vi "Rio_Main.vi"() -> ()   [LabVIEW 2017]
doc: "The myRIO Project template acquires acceleration data from the onboard accelerometer and displays the changes of acceleration values in a waveform chart."
uses:
  rio_states.ctl
  <vilib>/myRIO/Common/Instrument Driver Framework/myRIO v1.0/Encoder/typedefs/Encoder Signal Mode.ctl
  <vilib>/myRIO/Instrument Drivers/Onboard IO/Encoder/typedefs/Encoder Reference.ctl
  <vilib>/myRIO/Common/Instrument Driver Framework/Utilities/typedefs/myRIO Generic Hardware Reference.ctl
  <vilib>/myRIO/Common/Instrument Driver Framework/Utilities/typedefs/Hardware Version Enum.ctl
  <vilib>/myRIO/Common/Instrument Driver Framework/Utilities/typedefs/myRIO v1.0 Reference.ctl
  <vilib>/myRIO/Common/Instrument Driver Framework/Utilities/typedefs/Generic FPGA Reference.ctl
  <vilib>/myRIO/Common/Instrument Driver Framework/myRIO v1.0/Encoder/typedefs/Encoder Channels Enum.ctl
  <vilib>/myRIO/Common/Instrument Driver Framework/myRIO v1.0/Encoder/typedefs/Encoder Configuration v1.0.ctl
  <vilib>/userdefined/High Color/nirio_resource_hc.ctl
  <vilib>/myRIO/Common/Instrument Driver Framework/Utilities/vis/Is FPGA Ref Available.vi
  <vilib>/myRIO/Common/Instrument Driver Framework/myRIO v1.0/Encoder/vis/myRIO v1.1 Open Encoder.vi
  <vilib>/myRIO/Instrument Drivers/Onboard IO/Encoder/vis/Read.vi
  <vilib>/myRIO/Common/Instrument Driver Framework/Utilities/vis/Validate Channels.vi
  <vilib>/myRIO/Common/Instrument Driver Framework/myRIO v1.0/Encoder/vis/myRIO v1.0 Reserve Encoder.vi
  <vilib>/myRIO/Common/Instrument Driver Framework/myRIO v1.0/Encoder/vis/myRIO v1.0 Build MUX Configuration Encoder.vi
  <vilib>/myRIO/Common/Instrument Driver Framework/myRIO v1.0/Resource Manager/vis/myRIO v1.0 Reserve Channel List.vi
  <vilib>/myRIO/Common/Instrument Driver Framework/myRIO v1.0/Resource Manager/vis/myRIO v1.0 Create Configuration List.vi
  <vilib>/myRIO/Common/Instrument Driver Framework/myRIO v1.0/Resource Manager/vis/myRIO v1.0 Reserve Channel.vi
  <vilib>/myRIO/Common/Instrument Driver Framework/myRIO v1.0/Resource Manager/vis/myRIO v1.0 Unreserve Channel.vi
  <vilib>/myRIO/Common/Instrument Driver Framework/myRIO v1.0/Resource Manager/vis/myRIO v1.0 Build Mutex Name.vi
  <vilib>/Utility/VariantDataType/GetNumericInfo.vi
  <vilib>/Utility/error.llb/Error Cluster From Error Code.vi
  <vilib>/myRIO/Common/Instrument Driver Framework/myRIO v1.0/myRIO v1.1 Open.vi
  <vilib>/myRIO/Common/Instrument Driver Framework/Utilities/vis/IO Manager.vi
  <vilib>/myRIO/Common/Instrument Driver Framework/Utilities/vis/Configuration Manager.vi
  <vilib>/myRIO/Common/Instrument Driver Framework/myRIO v1.0/Resource Manager/vis/myRIO v1.0 Configure IO.vi
  <vilib>/myRIO/Common/Instrument Driver Framework/myRIO v1.0/myRIO v1.0 Close.vi
  <vilib>/myRIO/Common/Instrument Driver Framework/myRIO v1.0/Encoder/vis/myRIO v1.0 Configure Encoder.vi
  <vilib>/myRIO/Common/Instrument Driver Framework/myRIO v1.0/Encoder/vis/myRIO v1.0 Read Encoder.vi
  <vilib>/myRIO/Express VI/Onboard IO/Encoder/Encoder Express VI.xnode
  <vilib>/myRIO/Instrument Drivers/Onboard IO/Encoder/vis/myRIO Encoder Open.xnode
  <vilib>/myRIO/Common/Instrument Driver Framework/myRIO v1.0/Encoder/typedefs/Encoder Count Direction Enum.ctl
  <vilib>/myRIO/Instrument Drivers/Onboard IO/Encoder/Encoder.lvlib
panel:
  in  "Array":dbl[][](array[numeric]) format="%#_13g"
  in  "stop":bool
  out "Y Encoder":i32
  out "Y Encoder":i32
  in  "rio_states":T1
  out "String":string
  in  "Calibrate XY":bool
  out "Error Out":errorcluster
  in  "Error In":errorcluster
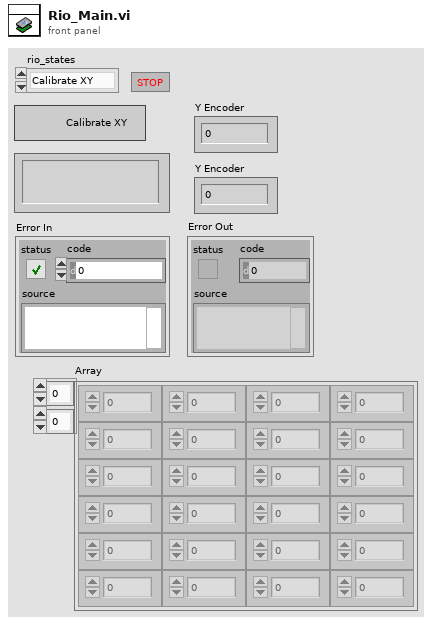
[diagram p1: front panel]
types:
  T1 = typedef "rio_states.ctl" = enum16{"Calibrate XY", "Move Theta", "Move XY", "Collect Kicker", "Pickup Kicker", "Retract Kicker", "Hold Kicker", "Kick", "Return Home", "Next Shot", "Stop"}
  T2 = typedef "rio_states.ctl" = cluster{enum16{"Calibrate XY", "Calibrate Theta", "Pickup Kicker", "Raise Kicker", "Move XY", "Move Theta", "Set Kicker Power", "Kick", "Stop"}, "Message Data":variant}
  T3 = enum16{"Calibrate XY", "Calibrate Theta", "Pickup Kicker", "Raise Kicker", "Move XY", "Move Theta", "Set Kicker Power", "Kick", "Stop"}
  T4 = typedef "Encoder.lvlib/Encoder Reference.ctl" = cluster{"myRIO Reference":T5, "Encoder Channels Enum":T9}
  T5 = typedef "myRIO Generic Hardware Reference.ctl" = cluster{"myRIO Model":T6, "myRIO Hardware Reference":T7}
  T6 = typedef "Hardware Version Enum.ctl" = enum16{"Unknown", "myRIO-1900", "myRIO-1950", "roboRIO", "NI ELVIS RIO CM"}
  T7 = typedef "myRIO v1.0 Reference.ctl" = cluster{"Generic FPGA Reference":T8, "Allow multiple opens":bool}
  T8 = typedef "Generic FPGA Reference.ctl" = refnum<k20>
  T9 = typedef "Encoder Channels Enum.ctl" = enum16{"Not Connected", "C/ENC0", "C/ENC1", "A/ENC", "B/ENC", "DIO/ENC0", "DIO/ENC1", "DIO/ENC2", "DIO/ENC3", "DIO/ENC4"}
  T10 = typedef "Encoder Signal Mode.ctl" = enum16{"Quadrature phase signal", "Step and direction signal"}
  T11 = typedef "nirio_resource_hc.ctl" = tag
  T12 = cluster{"Counter Value":i32, "Counter Value":i32}
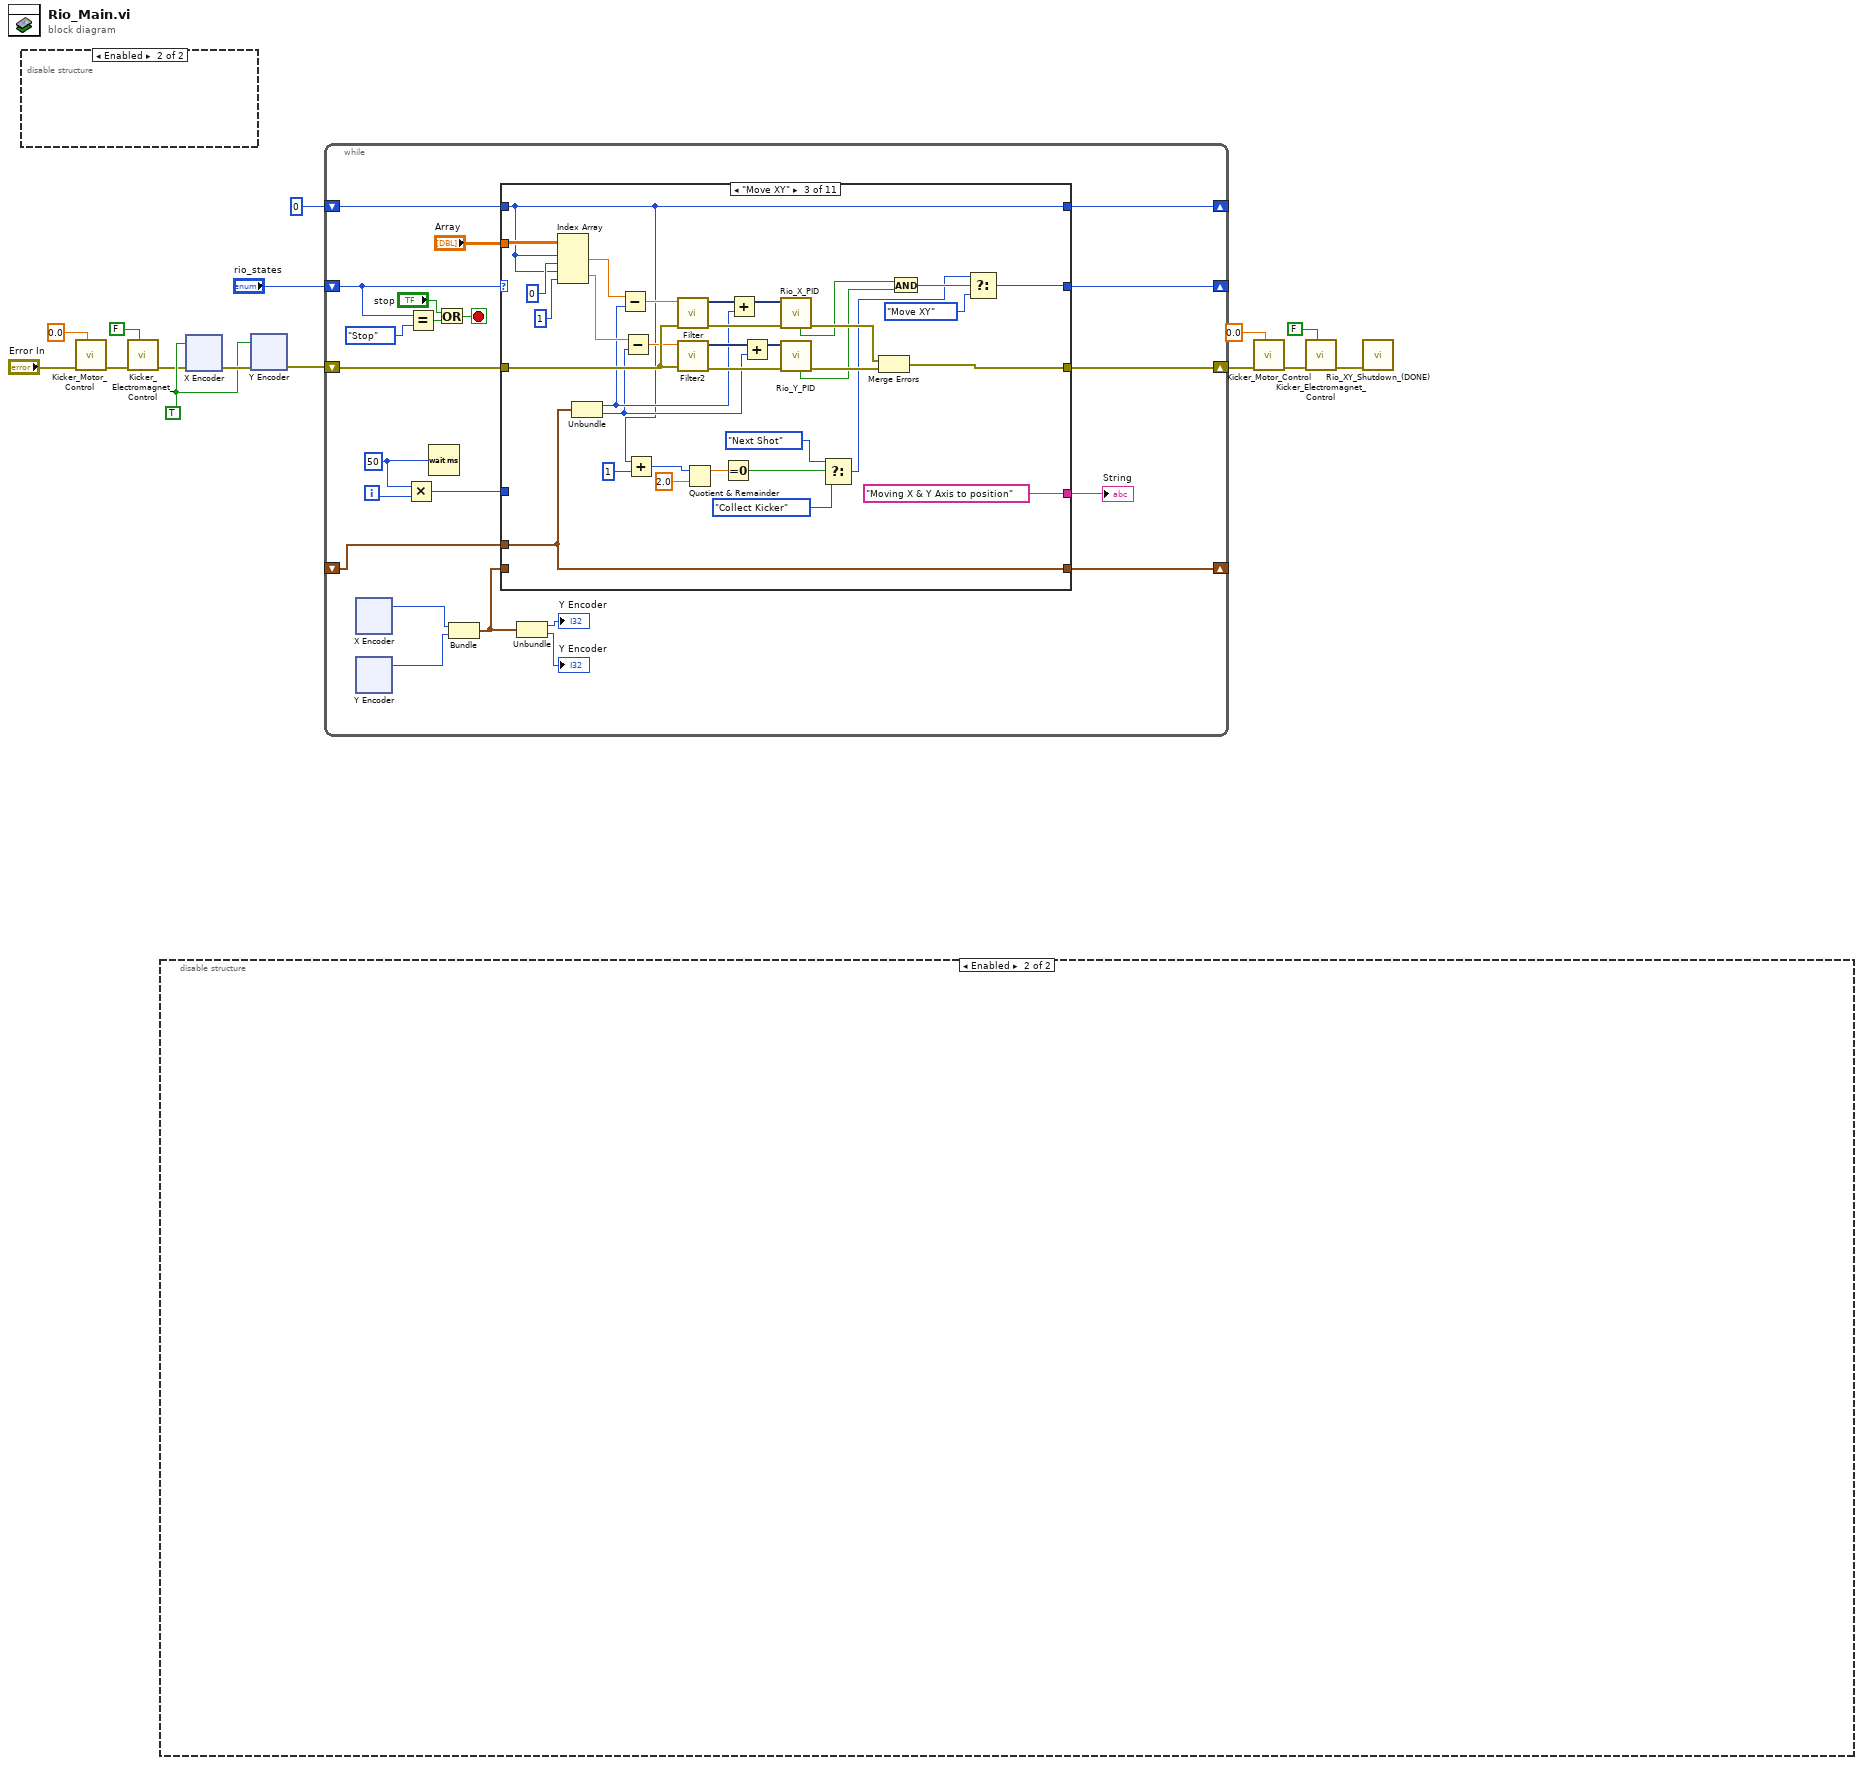
[diagram p0: block diagram]
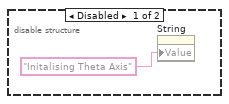
[diagram p2: hidden frame]
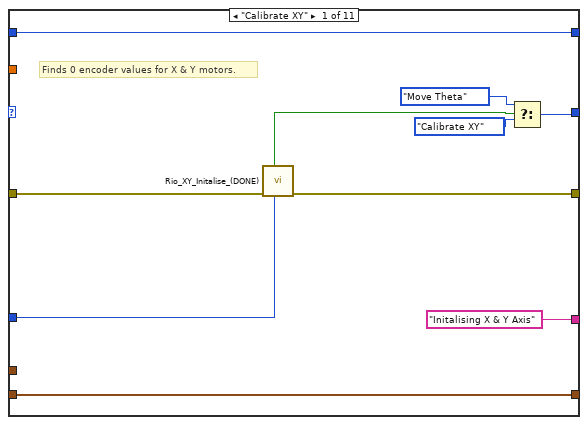
[diagram p3: hidden frame]
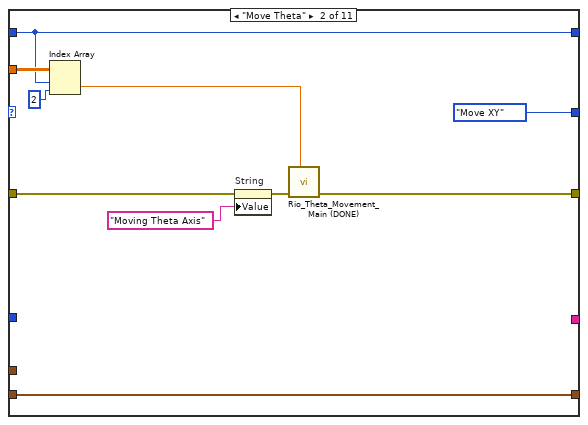
[diagram p4: hidden frame]
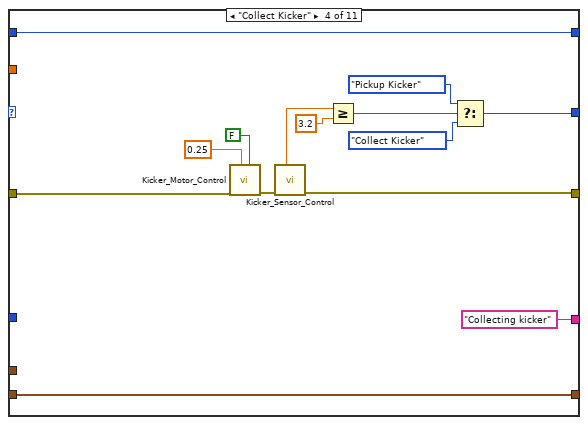
[diagram p5: hidden frame]
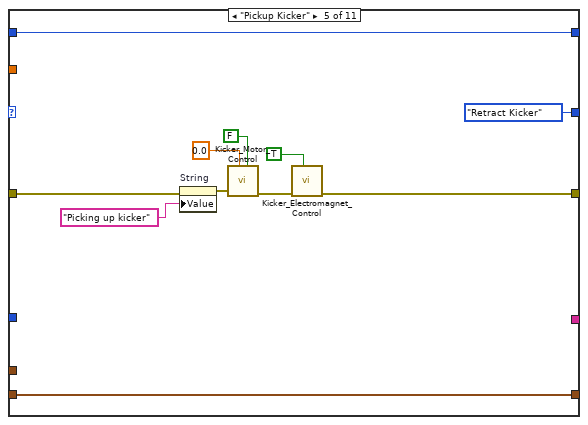
[diagram p6: hidden frame]
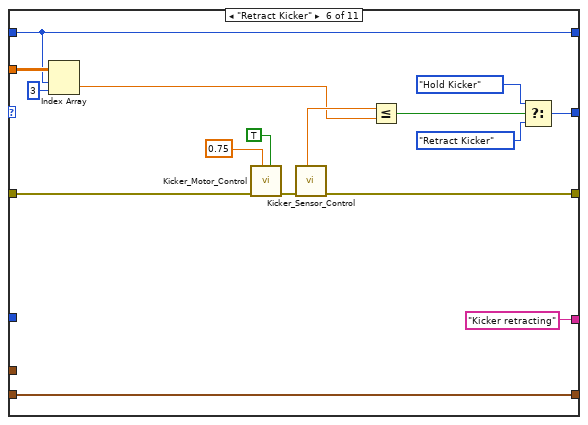
[diagram p7: hidden frame]
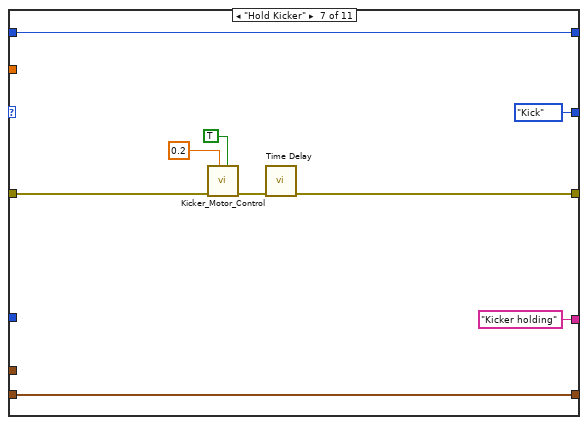
[diagram p8: hidden frame]
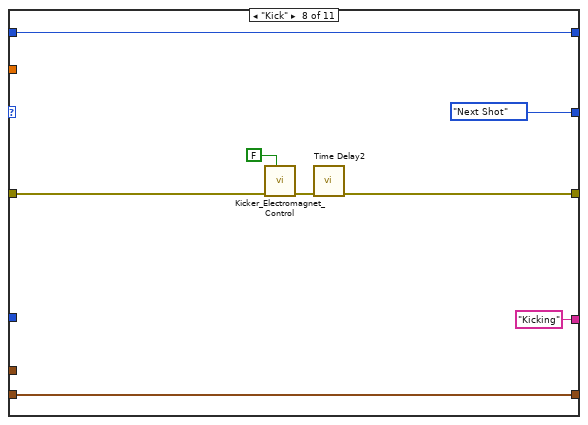
[diagram p9: hidden frame]
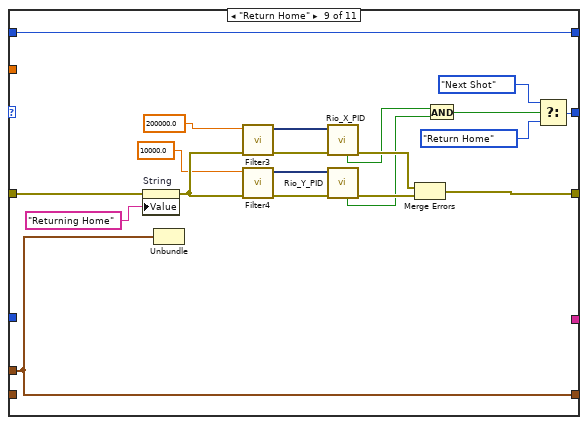
[diagram p10: hidden frame]
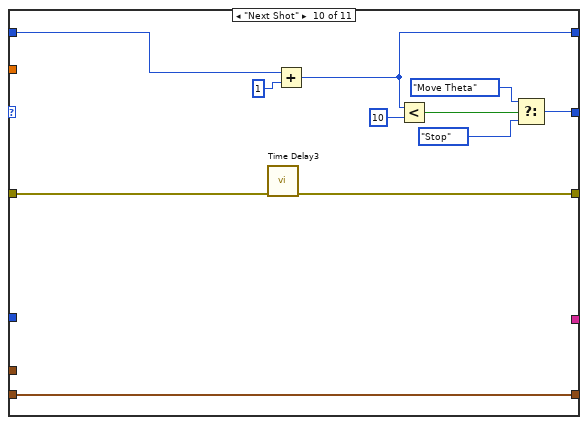
[diagram p11: hidden frame]
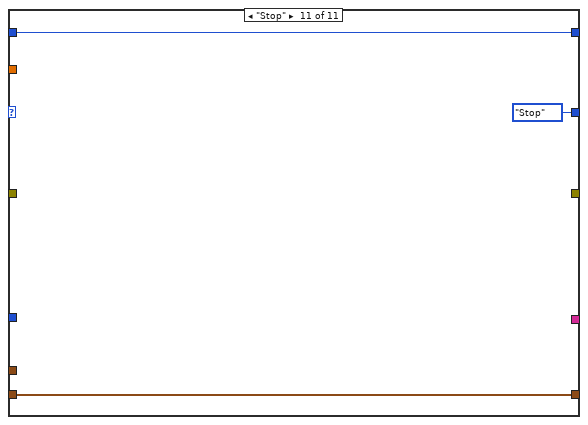
[diagram p12: hidden frame]
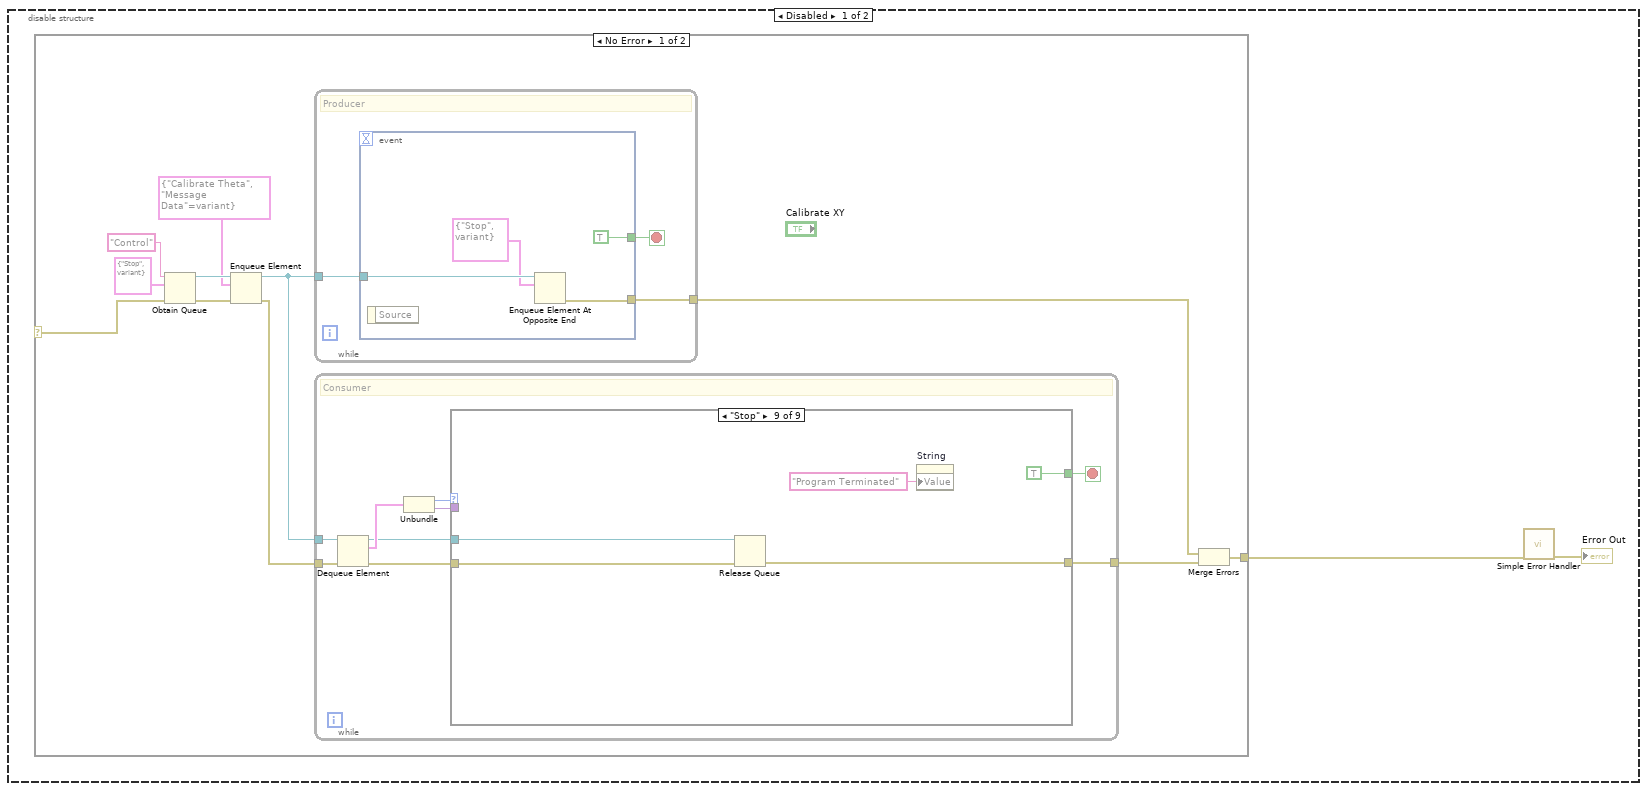
[diagram p13: hidden frame]
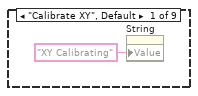
[diagram p14: hidden frame]
diagram:
  w12 = TRUE ("Reset Counter")
  n1 = disable-structure shown="Enabled" {
    frame Disabled {
      n2 = property on="String" class="Str"("Value"="Initalising Theta Axis" ("String")) -> ()  [unwired: 2 in, 2 out]
    }
    frame Enabled {
    }
  }
  n3 = call "Kicker_Motor_Control.vi"("Duty Cycle"=0.0, "error in"="Error In") -> ("error out"=w9:errorcluster)  [unwired: 9 in]
  n4 = call "Kicker_Electromagnet_Control.vi"("Mag Enable"=FALSE, "error in"=w9) -> ("error out"=w8:errorcluster)  [unwired: 9 in]
  n5 = disable-structure shown="Enabled" {
    frame Disabled {
      n6 = case shown="No Error" w17 {
        selector: [w22 w53] -> w17
        tunnel: [w30 w53] -> w18
        frame No Error {
          n7 = Obtain Queue(name (unnamed)="Control", element data type=T2 {enum."Stop", "Message Data"=variant}, error in (no error)=w22) -> (queue out=w24:refnum<queue>, error out=w25:errorcluster)  [unwired: 2 in, 1 out]
          n8 = Enqueue Element(queue=w24, element=T2 {enum."Calibrate Theta", "Message Data"=variant}, error in (no error)=w25) -> (queue out=w21:refnum<queue>, error out=w20:errorcluster)  [unwired: 1 in, 1 out]
          n9 = while {
            tunnel: [w47] -> w29
            tunnel: w21 -> [w48]
            stop <- w46 stop-if-true
            # "Producer"
            n10 = event {
              selector: _ -> [_]
              dyn-events: _ -> [_]
              timeout: _ -> [_]
              tunnel: w48 -> [w52]
              tunnel: [w51] -> w47
              tunnel: [TRUE] -> w46
              event #0 {
                n11 = event-data() -> ()  [unwired: 1 in, 1 out]
                n12 = Enqueue Element At Opposite End(queue=w52, element=T2 {enum."Stop", "Message Data"=variant}) -> (error out=w51:errorcluster)  [unwired: 2 in, 2 out]
              }
            }
          }
          n13 = while {
            tunnel: w20 -> [w39]
            tunnel: [w34] -> w27
            tunnel: w21 -> [w31]
            stop <- w33 stop-if-true
            # "Consumer"
            n14 = Dequeue Element(queue=w31, error in (no error)=w39) -> (queue out=w35:refnum<queue>, element=w37:T2, error out=w38:errorcluster)  [unwired: 1 in, 1 out]
            n15 = Unbundle(w37) -> (w36:T3, "Message Data"=w32:variant)
            n16 = case shown="\"Stop\"" w36 {
              tunnel: w38 -> [_ _ _ _ _ _ _ _ w45]
              tunnel: w35 -> [_ _ _ _ _ _ _ _ w42]
              tunnel: [_ _ _ _ _ _ _ _ w44] -> w34
              tunnel: [_ _ _ _ _ _ _ _ TRUE] -> w33
              tunnel: w32 -> [_ _ _ _ _ _ _ _ _]
              frame "Calibrate XY", Default {
                n17 = property on="String" class="Str"("Value"="XY Calibrating" ("String")) -> ()  [unwired: 2 in, 2 out]
              }
              frame "Calibrate Theta" {
              }
              frame "Pickup Kicker" {
              }
              frame "Raise Kicker" {
              }
              frame "Move XY" {
              }
              frame "Move Theta" {
              }
              frame "Set Kicker Power" {
              }
              frame "Kick" {
              }
              frame "Stop" {
                n18 = Release Queue(queue=w42, error in (no error)=w45) -> (error out=w44:errorcluster)  [unwired: 1 in, 2 out]
                n19 = property on="String" class="Str"("Value"="Program Terminated" ("String")) -> ()  [unwired: 2 in, 2 out]
              }
            }
          }
          n20 = Merge Errors(w29, w27) -> (w30:errorcluster)
        }
        frame Error {
        }
      }
      n21 = call <vilib>:"Simple Error Handler.vi"("error in (no error)"=w18) -> ("error out"=→"Error Out":errorcluster)  [unwired: 4 in, 4 out]
    }
    frame Enabled {
    }
  }
  n22 = xnode "X Encoder"("error in (no error)"=w8, "Reset Counter"=w12) -> ("error out"=w14:errorcluster)  [unwired: 3 out]
  n23 = xnode "Y Encoder"("error in (no error)"=w14, "Reset Counter"=w12) -> ("error out"=w13:errorcluster)  [unwired: 3 out]
  n24 = while {
    shift-right: [w75] -> _
    shift-left: "rio_states" -> [w74]
    shift-right: [w69] -> w4
    shift-left: w13 -> [w70]
    shift-right: [w58] -> _
    shift-left: _ -> [w59]
    shift-right: [w55] -> _
    shift-left: 0 -> [w56]
    i -> [w67]
    stop <- w65 stop-if-true
    w68 = u32 50 ("milliseconds to wait")
    n25 = xnode "X Encoder"() -> ("Counter Value"=w63:i32)  [unwired: 2 in, 3 out]
    n26 = xnode "Y Encoder"() -> ("Counter Value"=w62:i32)  [unwired: 2 in, 3 out]
    n27 = Multiply(x=w68, y=w67) -> (x*y=w66:u32)
    n28 = Equal?(x=w74, y=rio_states."Stop" ("rio_states")) -> (x = y?=w73:bool)
    n29 = Wait (ms)(milliseconds to wait=w68) -> ()  [unwired: 1 out]
    n30 = Or(x="stop", y=w73) -> (x .or. y?=w65:bool)
    n31 = Bundle("Counter Value"=w63, "Counter Value"=w62) -> (w54:T12)  [unwired: 1 in]
    n32 = case shown="\"Move XY\"" w74 {
      tunnel: [w173 rio_states."Move XY" ("rio_states") w213 w228 rio_states."Retract Kicker" ("rio_states") w256 rio_states."Kick" ("rio_states") rio_states."Next Shot" ("rio_states") w290 w307 rio_states."Stop" ("rio_states")] -> w75
      tunnel: ["Initalising X & Y Axis" ("String") _ "Moving X & Y Axis to position" ("String") "Collecting kicker" ("String") _ "Kicker retracting" ("String") "Kicker holding" ("String") "Kicking" ("String") _ _ _] -> w71
      tunnel: w70 -> [w176 w184 w212 w236 w240 w254 w267 w279 w288 w304 _]
      tunnel: [w177 w185 w217 w232 w243 w259 w270 w276 w291 w303 _] -> w69
      tunnel: w66 -> [w175 _ _ _ _ _ _ _ _ _ _]
      tunnel: w54 -> [w168 w178 _ w224 w238 w252 w265 w274 _ w305 w313]
      tunnel: [w168 w178 w209 w224 w238 w252 w265 w274 w286 w305 w313] -> w58
      tunnel: w59 -> [_ _ w209 _ _ _ _ _ w286 _ _]
      tunnel: "Array" -> [_ w182 w208 _ _ w250 _ _ _ _ _]
      tunnel: w56 -> [w169 w180 w189 w223 w237 w248 w264 w273 w285 w302 w312]
      tunnel: [w169 w180 w189 w223 w237 w248 w264 w273 w285 w310 w312] -> w55
      frame "Calibrate XY" {
        # "Finds 0 encoder values for X & Y motors."
        n33 = call "Rio_XY_Initalise_(DONE).vi"("Time Passed"=w175, "Error In"=w176) -> ("Error Out"=w177:errorcluster, "Axis Initalised"=w170:bool)  [unwired: 8 in]
        n34 = Select(t=rio_states."Move Theta" ("rio_states"), s=w170, f=rio_states."Calibrate XY" ("rio_states")) -> (s? t:f=w173:T1)
      }
      frame "Move Theta" {
        n35 = Index Array(array=w182, index (row)=w180, index (col)=2 ("disabled index (col)")) -> (element=w179:dbl)
        n36 = property on="String" class="Str"(error in=w184, "Value"="Moving Theta Axis" ("String")) -> (error out=w187:errorcluster)  [unwired: 1 in, 1 out]
        n37 = call "Rio_Theta_Movement_Main (DONE).vi"("Desired Position"=w179, "Error In"=w187) -> ("error out"=w185:errorcluster)  [unwired: 9 in]
      }
      frame "Move XY" {
        n38 = Index Array(array=w208, index (row) #1=w189, index (col) #1=0 ("disabled index (col)"), index (row) #2=w189, index (col) #2=1 ("disabled index (col)")) -> (element #1=w205:dbl, element #2=w204:dbl)
        n39 = Unbundle(w209) -> ("Counter Value"=w199:i32, "Counter Value"=w197:i32)
        n40 = Subtract(x=w205, y=w199) -> (x-y=w202:dbl)
        n41 = Subtract(x=w204, y=w197) -> (x-y=w201:dbl)
        n42 = Add(x=w189, y=1) -> (x+y=w194:i32)
        n43 = call "Filter"("error in (no error)"=w212, "Signal"=w202) -> ("error out"=w221:errorcluster, "Filtered Signal"=w222:dynamicdata)  [unwired: 8 in]
        n44 = call "Filter2"("error in (no error)"=w212, "Signal"=w201) -> ("error out"=w220:errorcluster, "Filtered Signal"=w203:dynamicdata)  [unwired: 8 in]
        n45 = Quotient & Remainder(x=w194, y=2.0) -> (x-y*floor(x/y)=w193:dbl)  [unwired: 1 out]
        n46 = Equal To 0?(x=w193) -> (x = 0?=w192:bool)
        n47 = Add(x=w222, y=w199) -> (x+y=w200:dynamicdata)
        n48 = Add(x=w203, y=w197) -> (x+y=w198:dynamicdata)
        n49 = call "Rio_X_PID.vi"("Error In"=w221, "Setpoint"=w200) -> ("Error Out"=w219:errorcluster, "Stop"=w215:bool)  [unwired: 6 in, 2 out]
        n50 = call "Rio_Y_PID.vi"("Error In"=w220, "Setpoint"=w198) -> ("Error Out"=w218:errorcluster, "Stop"=w214:bool)  [unwired: 6 in, 2 out]
        n51 = Select(t=rio_states."Next Shot" ("rio_states"), s=w192, f=rio_states."Collect Kicker" ("rio_states")) -> (s? t:f=w188:T1)
        n52 = Merge Errors(w219, w218) -> (w217:errorcluster)
        n53 = And(x=w215, y=w214) -> (x .and. y?=w216:bool)
        n54 = Select(t=w188, s=w216, f=rio_states."Move XY" ("rio_states")) -> (s? t:f=w213:T1)
      }
      frame "Collect Kicker" {
        n55 = call "Kicker_Motor_Control.vi"("Motor Dir (T/F = U/D)"=FALSE ("Motor Dir"), "Duty Cycle"=0.25 ("Motor Speed"), "error in"=w236) -> ("error out"=w233:errorcluster)  [unwired: 8 in]
        n56 = call "Kicker_Sensor_Control.vi"("error in"=w233) -> ("error out"=w232:errorcluster, "Pot Output"=w230:dbl)  [unwired: 9 in]
        n57 = Greater Or Equal?(x=w230, y=3.2) -> (x >= y?=w229:bool)
        n58 = Select(t=rio_states."Pickup Kicker" ("rio_states"), s=w229, f=rio_states."Collect Kicker" ("rio_states")) -> (s? t:f=w228:T1)
      }
      frame "Pickup Kicker" {
        n59 = property on="String" class="Str"(error in=w240, "Value"="Picking up kicker" ("String")) -> (error out=w239:errorcluster)  [unwired: 1 in, 1 out]
        n60 = call "Kicker_Motor_Control.vi"("Motor Dir (T/F = U/D)"=FALSE ("Motor Dir"), "Duty Cycle"=0.0 ("Motor Speed"), "error in"=w239) -> ("error out"=w244:errorcluster)  [unwired: 8 in]
        n61 = call "Kicker_Electromagnet_Control.vi"("Mag Enable"=TRUE, "error in"=w244) -> ("error out"=w243:errorcluster)  [unwired: 9 in]
      }
      frame "Retract Kicker" {
        n62 = Index Array(array=w250, index (row)=w248, index (col)=3 ("disabled index (col)")) -> (element=w249:dbl)
        n63 = call "Kicker_Motor_Control.vi"("Motor Dir (T/F = U/D)"=TRUE ("Motor Dir"), "Duty Cycle"=0.75 ("Motor Speed"), "error in"=w254) -> ("error out"=w261:errorcluster)  [unwired: 8 in]
        n64 = call "Kicker_Sensor_Control.vi"("error in"=w261) -> ("error out"=w259:errorcluster, "Pot Output"=w260:dbl)  [unwired: 9 in]
        n65 = Less Or Equal?(x=w260, y=w249) -> (x <= y?=w255:bool)
        n66 = Select(t=rio_states."Hold Kicker" ("rio_states"), s=w255, f=rio_states."Retract Kicker" ("rio_states")) -> (s? t:f=w256:T1)
      }
      frame "Hold Kicker" {
        n67 = call "Kicker_Motor_Control.vi"("Motor Dir (T/F = U/D)"=TRUE ("Motor Dir"), "Duty Cycle"=0.2 ("Motor Speed"), "error in"=w267) -> ("error out"=w266:errorcluster)  [unwired: 8 in]
        n68 = call "Time Delay"("error in (no error)"=w266) -> ("error out"=w270:errorcluster)  [unwired: 10 in]
      }
      frame "Kick" {
        n69 = call "Kicker_Electromagnet_Control.vi"("Mag Enable"=FALSE, "error in"=w279) -> ("error out"=w277:errorcluster)  [unwired: 9 in]
        n70 = call "Time Delay2"("error in (no error)"=w277) -> ("error out"=w276:errorcluster)  [unwired: 10 in]
      }
      frame "Return Home" {
        n71 = property on="String" class="Str"(error in=w288, "Value"="Returning Home" ("String")) -> (error out=w287:errorcluster)  [unwired: 1 in, 1 out]
        n72 = Unbundle(w286) -> ()  [unwired: 2 out]
        n73 = call "Filter3"("error in (no error)"=w287, "Signal"=200000.0) -> ("error out"=w300:errorcluster, "Filtered Signal"=w281:dynamicdata)  [unwired: 8 in]
        n74 = call "Filter4"("error in (no error)"=w287, "Signal"=10000.0) -> ("error out"=w299:errorcluster, "Filtered Signal"=w282:dynamicdata)  [unwired: 8 in]
        n75 = call "Rio_X_PID.vi"("Error In"=w300, "Setpoint"=w281) -> ("Error Out"=w298:errorcluster, "Stop"=w295:bool)  [unwired: 6 in, 2 out]
        n76 = call "Rio_Y_PID.vi"("Error In"=w299, "Setpoint"=w282) -> ("Error Out"=w297:errorcluster, "Stop"=w294:bool)  [unwired: 6 in, 2 out]
        n77 = Merge Errors(w298, w297) -> (w291:errorcluster)
        n78 = And(x=w295, y=w294) -> (x .and. y?=w296:bool)
        n79 = Select(t=rio_states."Next Shot" ("rio_states"), s=w296, f=rio_states."Return Home" ("rio_states")) -> (s? t:f=w290:T1)
      }
      frame "Next Shot" {
        n80 = call "Time Delay3"("error in (no error)"=w304) -> ("error out"=w303:errorcluster)  [unwired: 10 in]
        n81 = Add(x=w302, y=1) -> (x+y=w310:i32)
        n82 = Less?(x=w310, y=10) -> (x < y?=w308:bool)
        n83 = Select(t=rio_states."Move Theta" ("rio_states"), s=w308, f=rio_states."Stop" ("rio_states")) -> (s? t:f=w307:T1)
      }
      frame "Stop" {
      }
    }
    "String" <- w71
    n84 = Unbundle(w54) -> ("Counter Value"=→"Y Encoder":i32, "Counter Value"=→"Y Encoder":i32)
  }
  n85 = call "Kicker_Motor_Control.vi"("Duty Cycle"=0.0, "error in"=w4) -> ("error out"=w6:errorcluster)  [unwired: 9 in]
  n86 = call "Kicker_Electromagnet_Control.vi"("Mag Enable"=FALSE, "error in"=w6) -> ("error out"=w2:errorcluster)  [unwired: 9 in]
  n87 = call "Rio_XY_Shutdown_(DONE).vi"("error in (no error)"=w2) -> ()  [unwired: 10 in, 1 out]
